vi "在字符串中显示多种字体.vi"() -> ()   [LabVIEW 2022 SP3]
doc: "本VI是为《我和LabVIEW》一书编写的示例。\n关于本书的介绍请参考网页：\nhttp://ruanqizhen.spaces.live.com/blog/cns!5852D4F797C53FB6!4310.entry"
panel:
  out "字符串":string
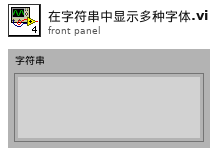
[diagram p1: front panel]
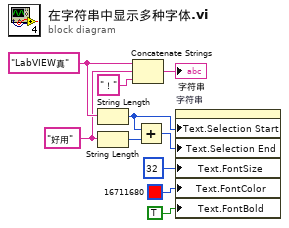
[diagram p0: block diagram]
diagram:
  w7 = "好用" ("字符串")
  w8 = "LabVIEW真" ("字符串")
  n1 = String Length(string=w8) -> (length=w4:i32)
  n2 = String Length(string=w7) -> (length=w6:i32)
  n3 = Concatenate Strings(w8, w7, "！" ("字符串")) -> (→"字符串":string)
  n4 = Add(x=w4, y=w6) -> (x+y=w5:i32)
  n5 = property on="字符串" class="Str"("Text.Selection Start"=w4, "Text.Selection End"=w5, "Text.FontSize"=u32 32 ("文本.字体:字号"), "Text.FontColor"=u32 16711680, "Text.FontBold"=TRUE ("文本.字体:粗体")) -> ()  [unwired: 2 in, 2 out]
